vi "Get Menu Items.vi"(8 "error in":errorcluster, 9 "GUID":string, 10 "Item Ref":T1 format="%.0x", 11 "System Explorer Dispatcher in":refnum<class "System Explorer Dispatcher.lvclass">) -> (0 "error out":errorcluster, 2 "Menu Items":cluster{"Name":string, "Enabled?":bool}[](array[cluster]), 3 "System Explorer Dispatcher out":refnum<class "System Explorer Dispatcher.lvclass">)   [LabVIEW 2020, in "AIM MIL-STD-1553 System Explorer.lvlib" / "Implementation.lvlib" / "System Explorer Dispatcher.lvclass"]
uses:
  System Explorer Dispatcher.lvclass
  Scripting/Constants.vi
  Scripting/AIM MIL-STD-1553 Scripting.lvlib
  <vilib>/NI VeriStand/Custom Device API/Custom Device Item Ref.ctl
  <vilib>/NI VeriStand/Custom Device API/Custom Device API.lvlib
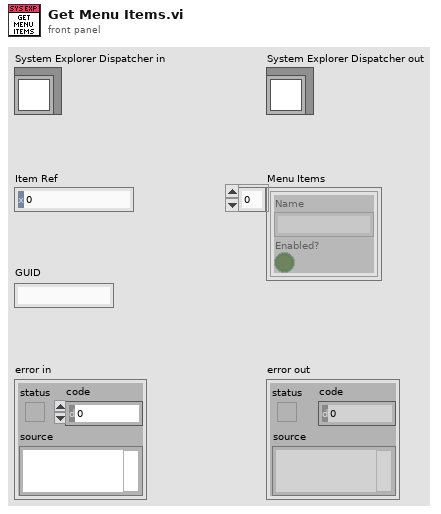
[diagram p1: front panel]
types:
  T1 = typedef "Custom Device API.lvlib/Custom Device Item Ref.ctl" = u64
  T2 = map{string, cluster{"Name":string, "Enabled?":bool}[]}
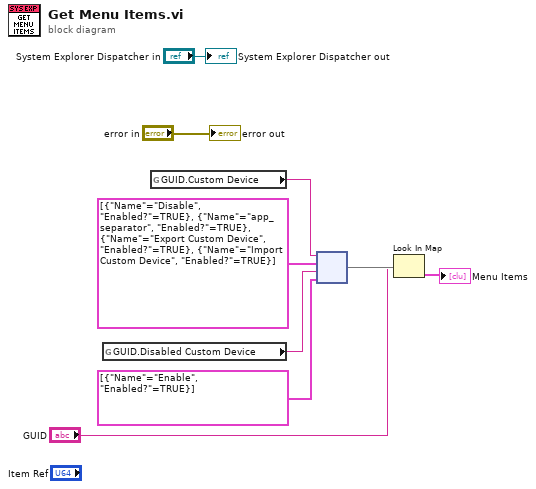
[diagram p0: block diagram]
diagram:
  n1 = global read "Constants.vi" "GUID.Disabled Custom Device"() -> (w2:string)
  n2 = global read "Constants.vi" "GUID.Custom Device"() -> (w7:string)
  n3 = node(w7, cluster{"Name":string, "Enabled?":bool}[] [{"Name"="Disable", "Enabled?"=TRUE}, {"Name"="app_separator", "Enabled?"=TRUE}, {"Name"="Export Custom Device", "Enabled?"=TRUE}, {"Name"="Import Custom Device", "Enabled?"=TRUE}] ("Menu Items"), w2, cluster{"Name":string, "Enabled?":bool}[] [{"Name"="Enable", "Enabled?"=TRUE}] ("Menu Items")) -> (w5:T2)
  n4 = Look In Map(map=w5, key="GUID") -> (value=→"Menu Items":cluster{"Name":string, "Enabled?":bool}[])  [unwired: 1 in, 1 out]
  "error out" <- "error in"
  "System Explorer Dispatcher out" <- "System Explorer Dispatcher in"
